vi "pic_step.vi"() -> ()   [LabVIEW 2018]
uses:
  Device VIs/Verbal.vi
  <vilib>/Instr/_visa.llb/VISA Configure Serial Port (Instr).vi
panel:
  in  "P3jog":bool caption="X jog"
  out "P3设定位置":i32
  in  "pic3位置":u16(ring) caption="位置" items=["位置0", "位置1", "位置2", "位置3"]
  in  "P3归0":bool
  in  "CH3启动":bool
  in  "CH3 运动步数":i32 caption="P3 步进"
  in  "Y 连续正转":bool
  in  "X连续反转":bool
  out "Yflag":bool
  out "0位":u8
  in  "P2 jog":bool caption="X jog"
  in  "P1jog":bool caption="X jog"
  in  "Zjog":bool caption="X jog"
  in  "Yjog":bool caption="X jog"
  in  "X jog":bool
  out "P2设定位置":i32
  out "P1设定位置":i32
  out "Z设定位置":i32
  out "Y设定位置":i32
  out "X设定位置":i32
  in  "pic2位置":u16(ring) caption="位置" items=["位置0", "位置1", "位置2", "位置3"]
  in  "pic1位置":u16(ring) caption="位置" items=["位置0", "位置1", "位置2", "位置3"]
  in  "Z轴位置":u16(ring) caption="位置" items=["位置0", "位置1", "位置2", "位置3"]
  in  "Y轴位置":u16(ring) caption="位置" items=["位置0", "位置1", "位置2", "位置3"]
  in  "X轴位置":u16(ring) caption="位置" items=["位置0", "位置1", "位置2", "位置3"]
  out "error in (no error)":errorcluster
  out "执行":bool
  in  "Z 归0":bool
  in  "Y 归0":bool
  in  "X 归0":bool
  out "当前位置":string[](array[string])
  in  "Z 连续反转":bool
  in  "Z 连续正转":bool
  in  "Y 连续反转":bool
  in  "X 连续正转":bool
  out "Z Left":bool caption="0位"
  out "Z Right":bool caption="限位"
  out "Y Left":bool caption="0位"
  out "Y Right":bool caption="限位"
  out "X Lift":bool caption="0位"
  out "X Right":bool caption="限位"
  in  "Z 启动":bool
  in  "Y 启动":bool
  in  "X 启动":bool
  in  "Step Z":i32 caption="Z 步进" min=-8388607 max=8388607
  in  "Step Y":i32 caption="Y 步进" min=-8388607 max=8388607
  in  "Step X":i32 caption="X 步进" min=-8388607 max=8388607
  in  "P2归0":bool
  in  "P1 归0":bool
  out "OK":bool
  in  "制动":bool
  in  "CH2启动":bool
  in  "CH1启动":bool
  in  "CH2 运动步数":i32 caption="P2 步进"
  in  "CH1 运动步数":i32 caption="P1 步进"
  out "CH2 当前位置":i32
  out "CH1 当前位置":i32
  out "状态":string
  out "error out":errorcluster
  # "X"
  # "Y"
  # "Z"
  # "P1"
  # "P2"
  # "P3"
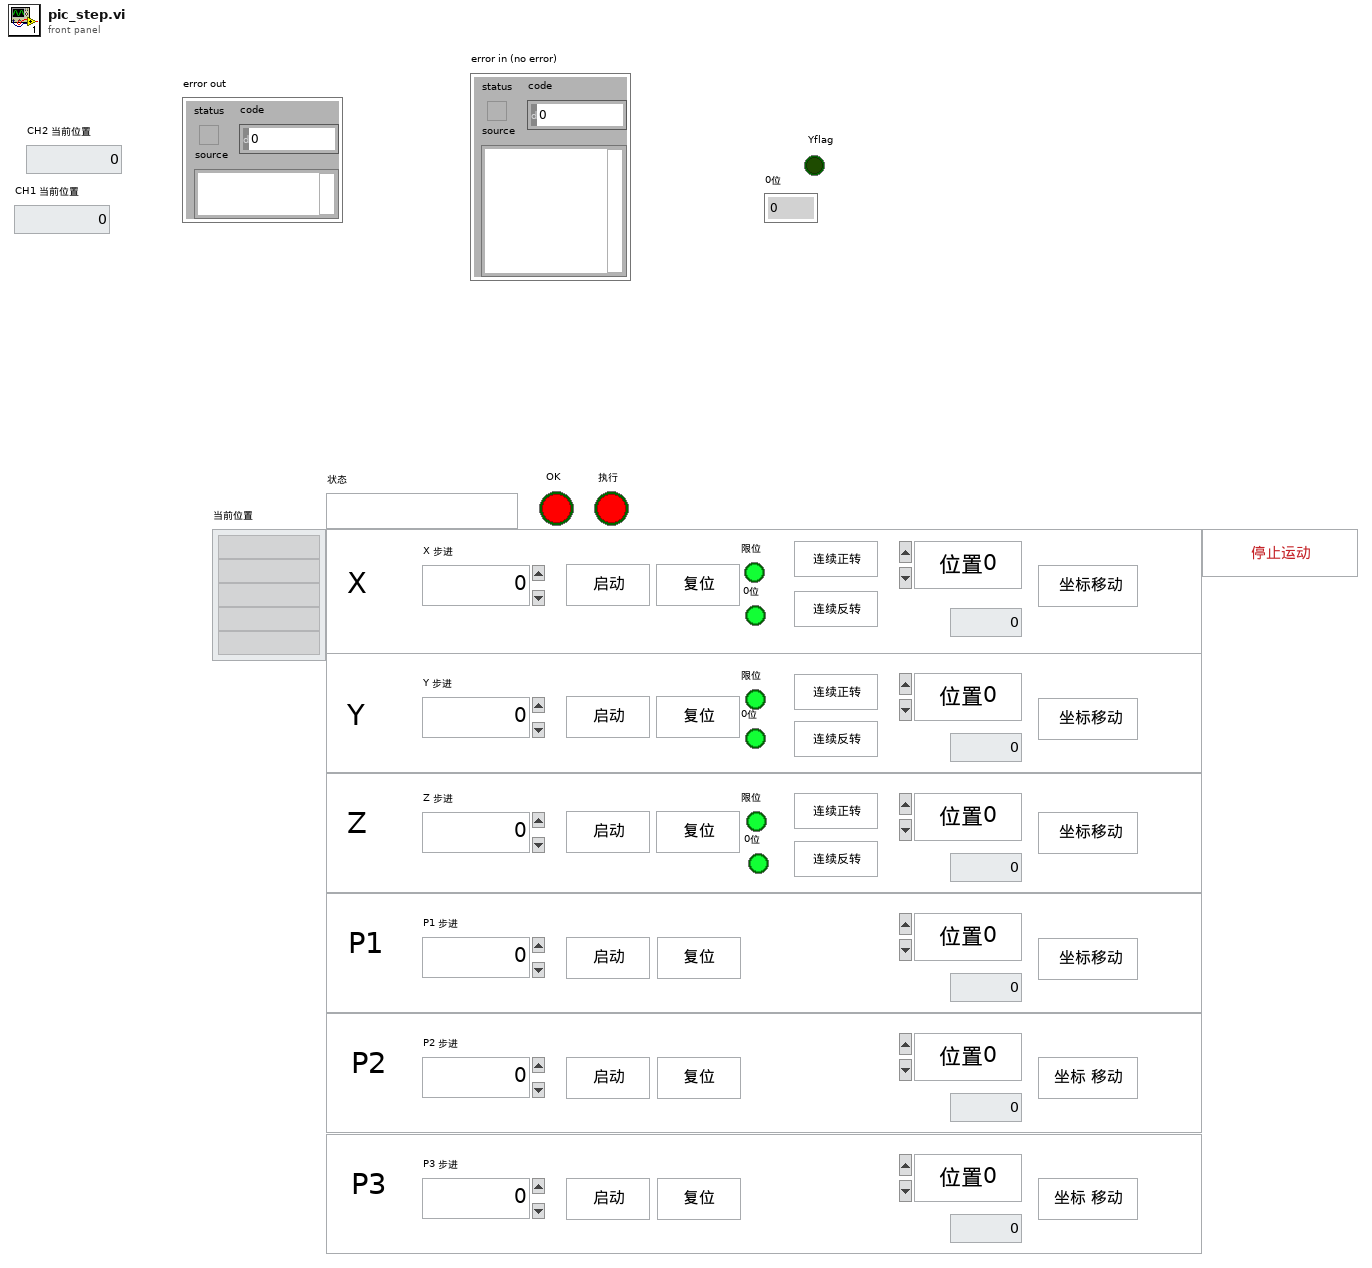
[diagram p1: front panel]
types:
  T1 = cluster{"DeviceKey":string, "Device Address":i32, "Controller Name":string}[]
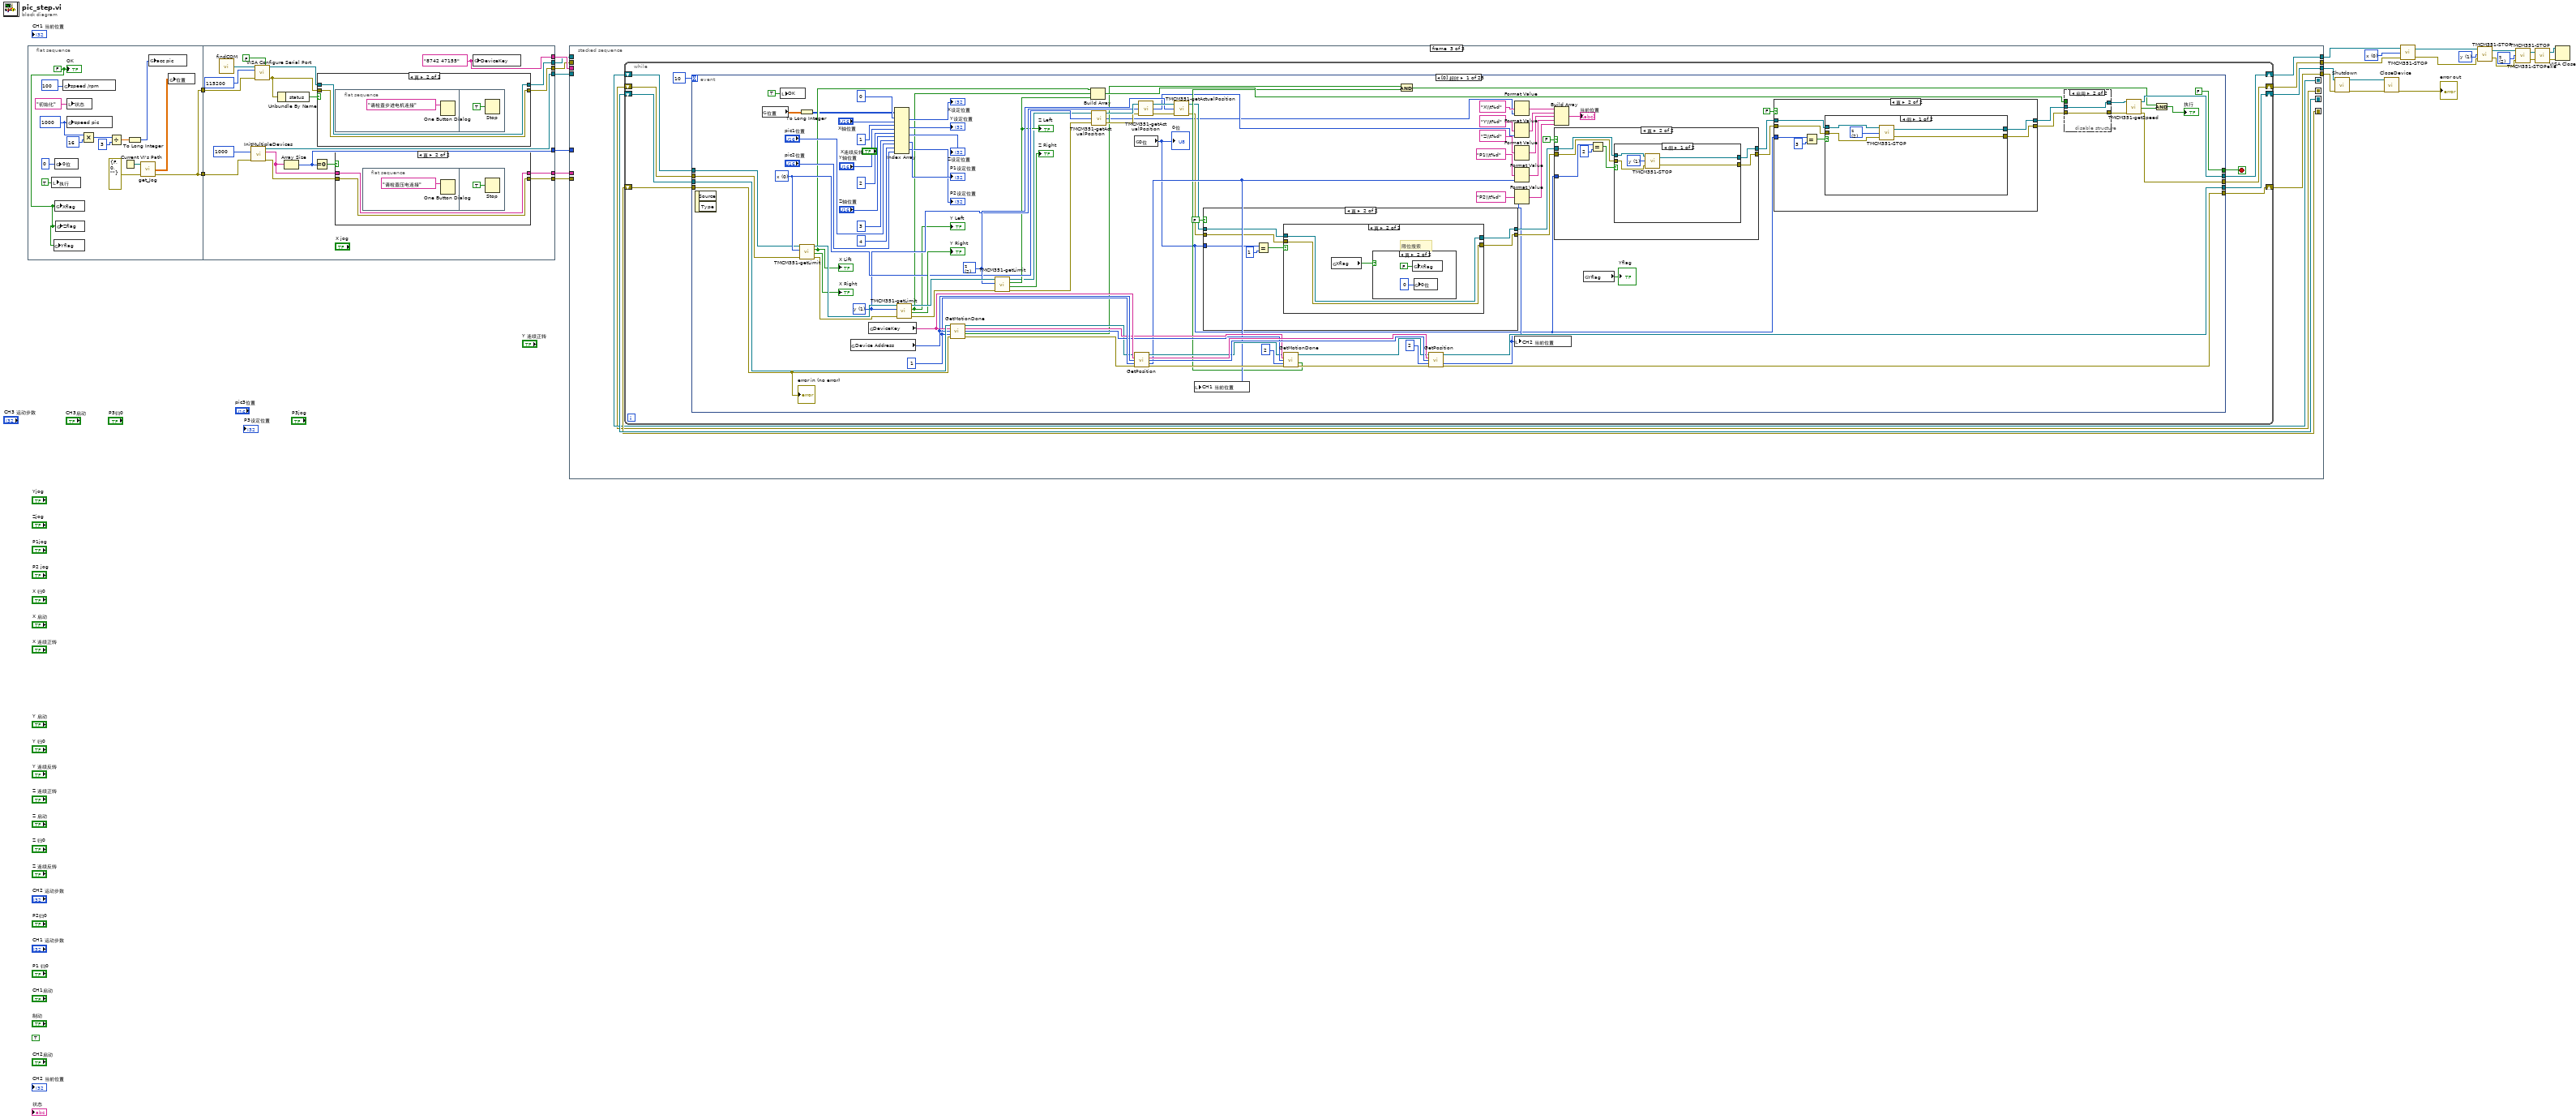
[diagram p0: block diagram]
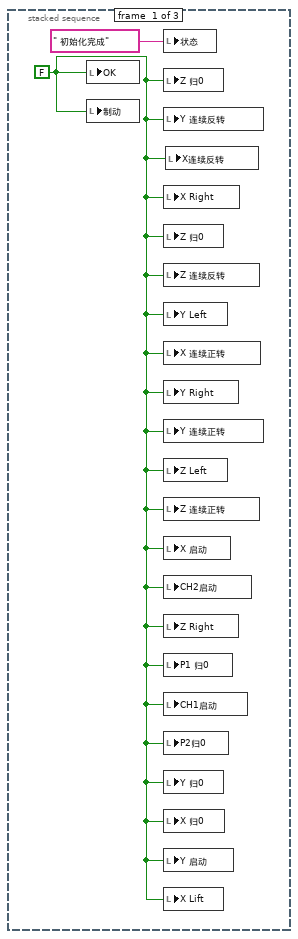
[diagram p4: hidden frame]
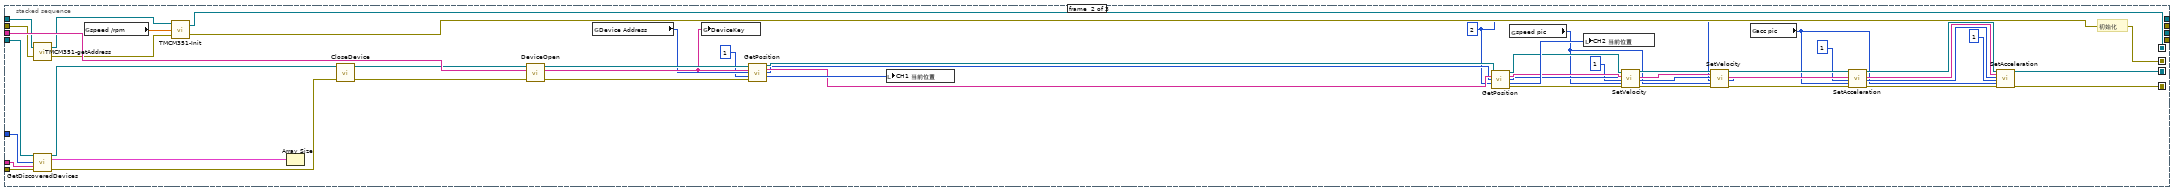
[diagram p5: hidden frame]
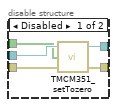
[diagram p6: hidden frame]
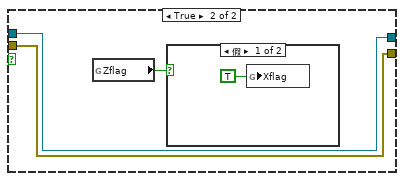
[diagram p8: hidden frame]
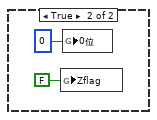
[diagram p9: hidden frame]
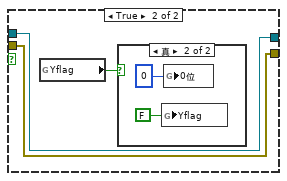
[diagram p11: hidden frame]
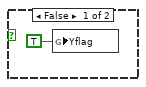
[diagram p12: hidden frame]
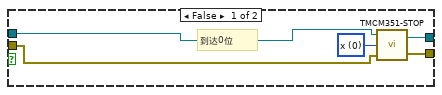
[diagram p14: hidden frame]
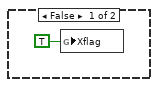
[diagram p15: hidden frame]
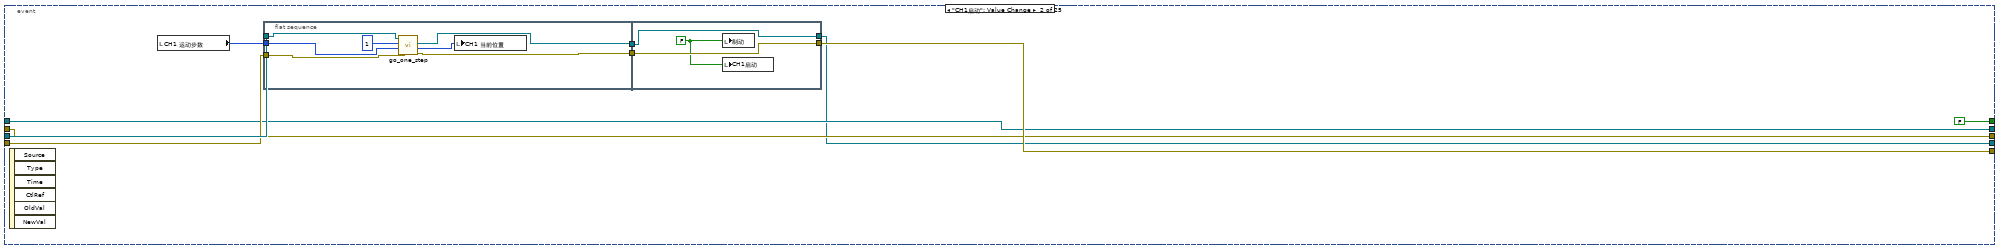
[diagram p16: hidden frame]
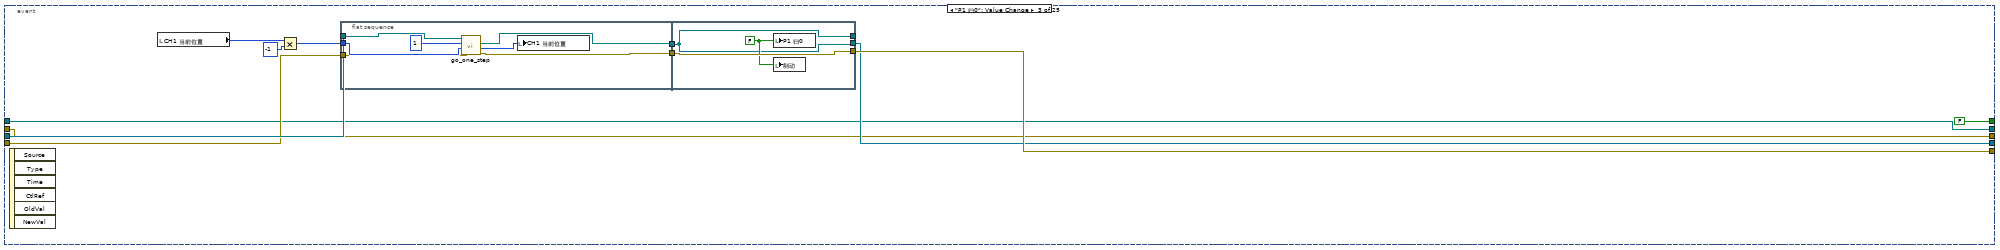
[diagram p17: hidden frame]
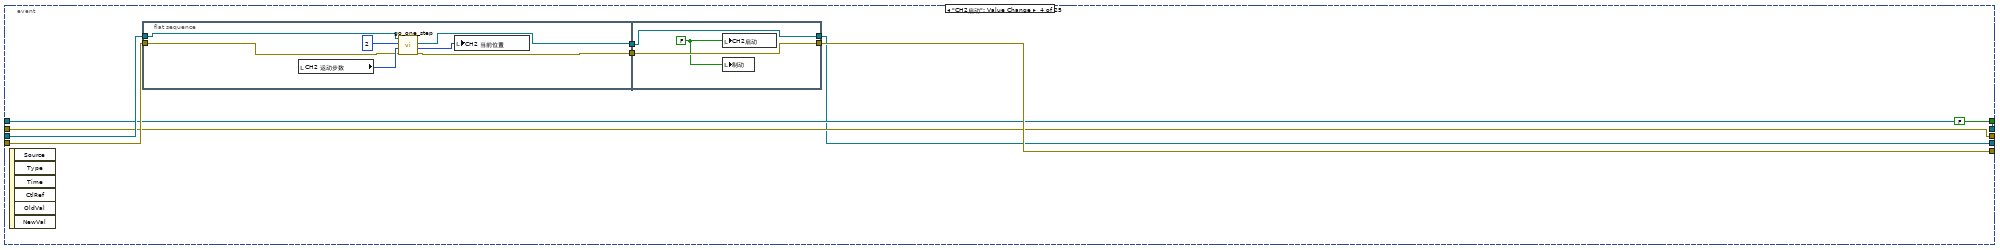
[diagram p18: hidden frame]
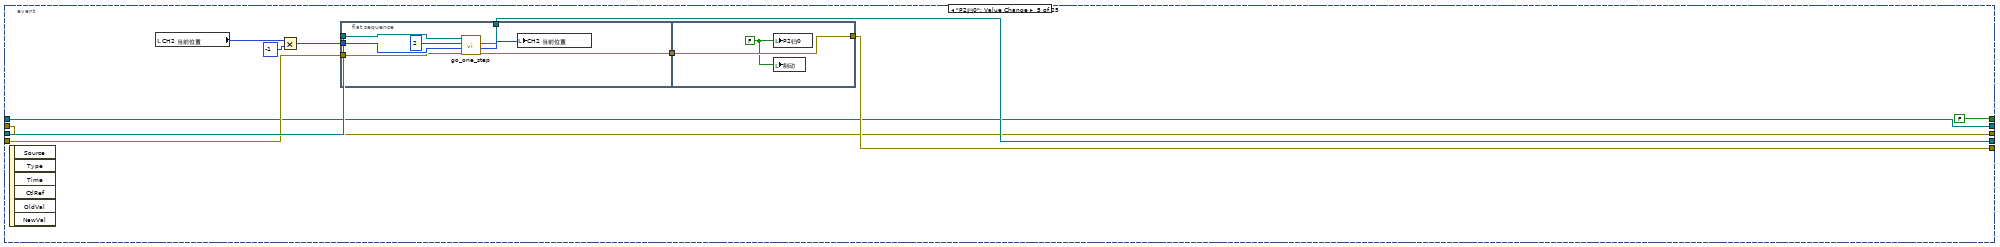
[diagram p19: hidden frame]
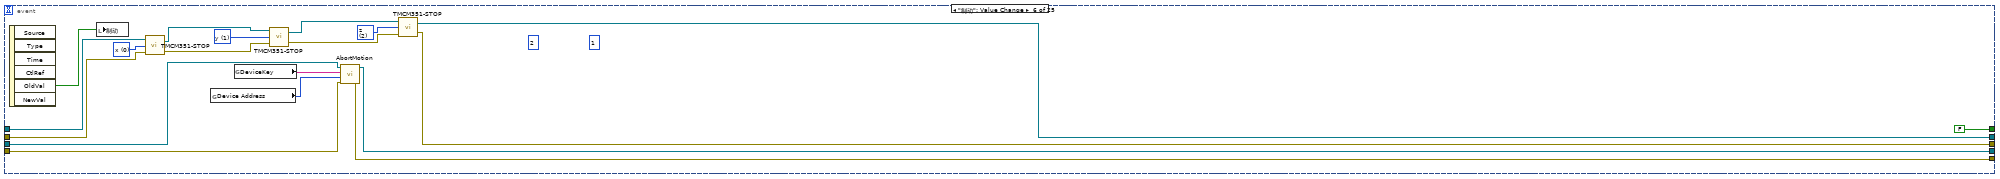
[diagram p20: hidden frame]
diagram:
  w10 = u8 2 items=["x", "y", "z"] ("motor")
  w11 = u8 1 items=["x", "y", "z"] ("motor")
  w12 = u8 0 items=["x", "y", "z"] ("motor")
  (unwired) TRUE
  n1 = flat-sequence {
    tunnel: [w31] -> w2
    tunnel: [w31] -> w1
    tunnel: [w61] -> w27
    tunnel: [w53] -> w26
    tunnel: [w52] -> w25
    tunnel: [w50] -> w24
    tunnel: [w49] -> w23
    tunnel: [w46] -> w22
    tunnel: [w45] -> w21
    tunnel: w2 -> [w44]
    tunnel: w1 -> [w43]
    frame #0 {
      w28 = FALSE ("OK")
      w37 = 1000 ("speed pic")
      n2 = local write "执行"(TRUE ("执行")) -> ()
      n3 = global write "Verbal.vi" "Yflag"(w28) -> ()
      n4 = global write "Verbal.vi" "0位"(u8 0 ("0位")) -> ()
      n5 = global write "Verbal.vi" "Xflag"(w28) -> ()
      n6 = global write "Verbal.vi" "Zflag"(w28) -> ()
      n7 = global write "Verbal.vi" "speed /rpm"(100 ("speed step")) -> ()
      n8 = local write "状态"("初始化" ("状态")) -> ()
      n9 = global write "Verbal.vi" "speed pic"(w37) -> ()
      n10 = Multiply(x=w37, y=u16 16) -> (x*y=w39:i32)
      n11 = Divide(x=w39, y=u16 3) -> (x/y=w36:dbl)
      n12 = Current VI's Path() -> (path=w33:path)
      n13 = To Long Integer(number=w36) -> (32bit integer=w35:i32)
      n14 = call "get_Jog.vi"("error in (no error)"=errorcluster {"status"=FALSE, "code"=0, "source"=""}, "路径"=w33) -> ("error out"=w31:errorcluster, "位置out"=w30:dbl[][])  [unwired: 2 in]
      n15 = global write "Verbal.vi" "acc pic"(w35) -> ()
      n16 = global write "Verbal.vi" "位置"(w30) -> ()
      "OK" <- w28
    }
    frame #1 {
      w61 = "8742 47155" ("Message")
      n17 = call "findCOM.vi"() -> ("VISA resource out"=w58:refnum<visa-resource-name>)  [unwired: 1 in]
      n18 = call "InitMultipleDevices.vi"("error in (no error)"=w43, "msecDelayForDiscovery"=1000) -> ("error out"=w47:errorcluster, "DeviceKey List Out"=w48:string[], "CmdLib Out"=w53:refnum<k24>)  [unwired: 3 in]
      n19 = call-poly "VISA Configure Serial Port"("VISA resource name"=w58, "Enable Termination\nChar (T)"=FALSE ("Enable Termination\nChar (T)"), "baud rate (9600)"=u32 115200, "error in (no error)"=w44) -> ("VISA resource name out"=w57:refnum<visa-resource-name>, "error out"=w55:errorcluster)  [unwired: 10 in]
      n20 = Unbundle By Name(w55) -> ("status"=w56:bool)
      n21 = Array Size(array=w48) -> (size(s)=w52:i32)
      n22 = Equal To 0?(x=w52) -> (x = 0?=w51:bool)
      n23 = case shown="真" w56 {
        tunnel: w57 -> [w69 w71]
        tunnel: w55 -> [w68 w70]
        tunnel: [w69 w71] -> w45
        tunnel: [w68 w70] -> w46
        frame False {
        }
        frame True {
          n24 = flat-sequence {
            frame #0 {
              n25 = One Button Dialog(message="请检查步进电机连接" ("消息")) -> ()  [unwired: 1 in, 1 out]
            }
            frame #1 {
              n26 = Stop(stop? (T)=TRUE ("停止？(T)")) -> ()
            }
          }
        }
      }
      n27 = case shown="真" w51 {
        tunnel: [w63 w65] -> w50
        tunnel: [w62 w64] -> w49
        tunnel: w48 -> [w63 w65]
        tunnel: w47 -> [w62 w64]
        frame False {
        }
        frame True {
          n28 = flat-sequence {
            frame #0 {
              n29 = One Button Dialog(message="请检查压电连接" ("消息")) -> ()  [unwired: 1 in, 1 out]
            }
            frame #1 {
              n30 = Stop(stop? (T)=TRUE ("停止？(T)")) -> ()
            }
          }
        }
      }
      n31 = global write "Verbal.vi" "DeviceKey"(w61) -> ()
    }
  }
  n32 = stacked-sequence {
    seq-local: [_ w79 _] -> [_ _ w134]
    seq-local: [_ w78 _] -> [_ _ w132]
    seq-local: [_ w119 _] -> [_ _ w131]
    seq-local: [_ w118 _] -> [_ _ w130]
    tunnel: w27 -> [_ w126 _]
    tunnel: [_ _ w133] -> w3
    tunnel: w25 -> [_ w125 _]
    tunnel: w24 -> [_ w124 _]
    tunnel: w26 -> [_ w123 _]
    tunnel: w23 -> [_ w122 _]
    tunnel: w22 -> [_ w121 _]
    tunnel: w21 -> [_ w120 _]
    tunnel: [_ _ w129] -> w14
    tunnel: [_ _ w128] -> w13
    tunnel: [_ _ w127] -> w4
    frame #0 {
      w74 = FALSE
      n33 = local write "OK"(w74) -> ()
      n34 = local write "制动"(w74) -> ()
      n35 = local write "状态"(" 初始化完成" ("Message")) -> ()
      n36 = local write "Z 归0"(w74) -> ()
      n37 = local write "Y 连续反转"(w74) -> ()
      n38 = local write "X Right"(w74) -> ()
      n39 = local write "Z 归0"(w74) -> ()
      n40 = local write "Z 连续反转"(w74) -> ()
      n41 = local write "Y Left"(w74) -> ()
      n42 = local write "X 连续正转"(w74) -> ()
      n43 = local write "Y Right"(w74) -> ()
      n44 = local write "Y 连续正转"(w74) -> ()
      n45 = local write "Z Left"(w74) -> ()
      n46 = local write "Z 连续正转"(w74) -> ()
      n47 = local write "X 启动"(w74) -> ()
      n48 = local write "CH2启动"(w74) -> ()
      n49 = local write "Z Right"(w74) -> ()
      n50 = local write "P1 归0"(w74) -> ()
      n51 = local write "CH1启动"(w74) -> ()
      n52 = local write "P2归0"(w74) -> ()
      n53 = local write "Y 归0"(w74) -> ()
      n54 = local write "X 归0"(w74) -> ()
      n55 = local write "Y 启动"(w74) -> ()
      n56 = local write "X Lift"(w74) -> ()
      n57 = local write "X连续反转"(w74) -> ()
    }
    frame #1 {
      w94 = 2 ("Motor")
      # "初始化"
      n58 = call "TMCM351-getAddress.vi"("错误输入"=w121, "com in"=w120) -> ("错误输出"=w92:errorcluster, "com out"=w77:refnum<visa-resource-name>)
      n59 = call "GetDiscoveredDevices.vi"("CmdLib In"=w123, "Master Count"=w125, "DeviceKey List"=w124, "error in"=w122) -> ("CmdLib Out"=w116:refnum<k24>, "Device Array"=w117:T1, "error out"=w114:errorcluster)  [unwired: 9 in]
      n60 = global read "Verbal.vi" "speed /rpm"() -> (w76:dbl)
      n61 = call "TMCM351-Init.vi"("错误输入"=w92, "Speed /rpm"=w76, "com in"=w77) -> ("错误输出"=w118:errorcluster, "com out"=w119:refnum<visa-resource-name>)
      n62 = Array Size(array=w117) -> ()  [unwired: 1 out]
      n63 = call "CloseDevice.vi"("error in"=w114, "CmdLib In"=w116) -> ("error out"=w113:errorcluster, "CmdLib Out"=w115:refnum<k24>)  [unwired: 8 in]
      n64 = call "DeviceOpen.vi"("error in (no error)"=w113, "DeviceKey In"=w126, "CmdLib In"=w115) -> ("error out"=w108:errorcluster, "DeviceKey Out"=w111:string, "CmdLib Out"=w112:refnum<k24>)  [unwired: 2 in]
      n65 = global read "Verbal.vi" "Device Address"() -> (w110:i32)
      n66 = global write "Verbal.vi" "DeviceKey"(w111) -> ()
      n67 = call "GetPosition.vi"("CmdLib In"=w112, "DeviceKey In"=w111, "Device Address In"=w110, "Motor"=1, "error in (no error)"=w108) -> ("CmdLib Out"=w106:refnum<k24>, "DeviceKey Out"=w105:string, "Device Address Out"=w104:i32, "Position"=w107:i32)  [unwired: 6 in, 1 out]
      n68 = local write "CH1 当前位置"(w107) -> ()
      n69 = call "GetPosition.vi"("CmdLib In"=w106, "DeviceKey In"=w105, "Device Address In"=w104, "Motor"=w94) -> ("CmdLib Out"=w102:refnum<k24>, "DeviceKey Out"=w101:string, "Device Address Out"=w100:i32, "Position"=w103:i32, "error out"=w98:errorcluster)  [unwired: 7 in]
      n70 = global read "Verbal.vi" "speed pic"() -> (w91:i32)
      n71 = local write "CH2 当前位置"(w103) -> ()
      n72 = call "SetVelocity.vi"("CmdLib In"=w102, "DeviceKey In"=w101, "Device Address In"=w100, "Motor"=1, "Steps Per Sec"=w91, "error in (no error)"=w98) -> ("CmdLib Out"=w97:refnum<k24>, "DeviceKey Out"=w96:string, "Device Address Out"=w95:i32, "error out"=w93:errorcluster)  [unwired: 10 in]
      n73 = call "SetVelocity.vi"("CmdLib In"=w97, "DeviceKey In"=w96, "Device Address In"=w95, "Motor"=w94, "Steps Per Sec"=w91, "error in (no error)"=w93) -> ("CmdLib Out"=w90:refnum<k24>, "DeviceKey Out"=w89:string, "Device Address Out"=w88:i32, "error out"=w86:errorcluster)  [unwired: 10 in]
      n74 = global read "Verbal.vi" "acc pic"() -> (w81:i32)
      n75 = call "SetAcceleration.vi"("CmdLib In"=w90, "DeviceKey In"=w89, "Device Address In"=w88, "Motor"=1, "Steps Per Sec 2"=w81, "error in (no error)"=w86) -> ("CmdLib Out"=w85:refnum<k24>, "DeviceKey Out"=w84:string, "Device Address Out"=w83:i32, "error out"=w80:errorcluster)  [unwired: 10 in]
      n76 = call "SetAcceleration.vi"("CmdLib In"=w85, "DeviceKey In"=w84, "Device Address In"=w83, "Motor"=1, "Steps Per Sec 2"=w81, "error in (no error)"=w80) -> ("CmdLib Out"=w79:refnum<k24>, "error out"=w78:errorcluster)  [unwired: 10 in, 2 out]
    }
    frame #2 {
      n77 = while {
        shift-right: [w142] -> w133
        shift-left: w132 -> [w140]
        shift-right: [w139] -> w127
        shift-left: w134 -> [w143]
        shift-right: [w138] -> w129
        shift-left: w131 -> [w136]
        shift-right: [w137] -> w128
        shift-left: w130 -> [w135]
        stop <- w141 stop-if-true
        n78 = event shown="[0] 超时" {
          selector: _ -> [_ _ _ _ _ _ _ _ _ _ _ _ _ _ _ _ _ _ _ _ _ _ _ _ _]
          dyn-events: _ -> [_ _ _ _ _ _ _ _ _ _ _ _ _ _ _ _ _ _ _ _ _ _ _ _ _]
          timeout: 10 -> [_ _ _ _ _ _ _ _ _ _ _ _ _ _ _ _ _ _ _ _ _ _ _ _ _]
          tunnel: w143 -> [w236 w318 w337 w359 w377 w406 w424 w440 w445 w458 w469 w484 w522 w561 w590 w601 w612 w623 w634 w645 w656 w666 w676 w694 w706]
          tunnel: w140 -> [w188 w317 w336 w357 w376 w407 w423 w439 w444 w457 w468 w483 w521 w560 w589 w600 w611 w622 w633 w644 w655 w665 w675 w689 w701]
          tunnel: [w237 w316 w334 w358 w375 w392 w422 w438 w444 w457 w468 w483 w521 w560 w589 w600 w611 w622 w633 w644 w655 w665 w675 w687 w699] -> w142
          tunnel: [FALSE FALSE FALSE FALSE FALSE FALSE TRUE TRUE FALSE FALSE FALSE FALSE FALSE _ _ _ _ _ _ _ _ _ _ _ _] -> w141
          tunnel: w136 -> [w164 w312 w330 w354 w371 w404 w413 w428 w450 w461 w473 w478 w514 w554 w599 w607 w618 w629 w640 w651 w662 w672 w682 w686 w698]
          tunnel: w135 -> [w163 w311 w329 w353 w370 w403 w412 w427 w449 w460 w471 w475 w513 w553 w598 w606 w617 w628 w639 w650 w661 w671 w681 w685 w697]
          tunnel: [w203 w309 w331 w351 w372 w391 w409 w436 w445 w458 w469 w484 w522 w561 w590 w601 w612 w623 w634 w645 w656 w666 w676 w688 w700] -> w139
          tunnel: [w185 w312 w330 w354 w371 w395 w411 w426 w447 w456 w467 w477 w520 w558 w594 w605 w616 w627 w638 w649 w660 w668 w678 w686 w698] -> w138
          tunnel: [w184 w311 w329 w353 w370 w394 w410 w425 w446 w455 w466 w476 w519 w559 w593 w604 w615 w626 w637 w648 w659 w667 w677 w685 w697] -> w137
          event Timeout {
            w210 = u8 2 items=["x", "y", "z"] ("motor")
            w191 = u8 1 items=["x", "y", "z"] ("motor")
            w192 = u8 0 items=["x", "y", "z"] ("motor")
            w233 = 1 ("Motor")
            n79 = event-data() -> ()  [unwired: 1 in, 2 out]
            n80 = global read "Verbal.vi" "位置"() -> (w159:dbl[][])
            n81 = local write "OK"(TRUE ("等待指令")) -> ()
            n82 = To Long Integer(number=w159) -> (32bit integer=w158:i32[][])
            n83 = call "TMCM351-getLimit.vi"("错误输入"=w163, "motor"=w192, "com in"=w164) -> ("错误输出"=w213:errorcluster, "right limit"=→"X Right":bool, "left limit"=w162:bool, "com out"=w214:refnum<visa-resource-name>)  [unwired: 1 in]
            "X Lift" <- w162
            n84 = global read "Verbal.vi" "Device Address"() -> (w234:i32)
            n85 = global read "Verbal.vi" "DeviceKey"() -> (w235:string)
            n86 = Index Array(array=w158, index (row) #1=0 ("索引 (行)"), index (col) #1="X轴位置", index (row) #2=1 ("索引 (行)"), index (col) #2="Y轴位置", index (row) #3=2 ("索引 (行)"), index (col) #3="Z轴位置", index (row) #4=3 ("索引 (行)"), index (col) #4="pic1位置", index (row) #5=4 ("索引 (行)"), index (col) #5="pic2位置") -> (element #1=→"X设定位置":i32, element #2=→"Y设定位置":i32, element #3=→"Z设定位置":i32, element #4=→"P1设定位置":i32, element #5=→"P2设定位置":i32)
            n87 = call "TMCM351-getLimit.vi"("错误输入"=w213, "motor"=w191, "com in"=w214) -> ("错误输出"=w211:errorcluster, "right limit"=→"Y Right":bool, "left limit"=w161:bool, "com out"=w212:refnum<visa-resource-name>)  [unwired: 1 in]
            "Y Left" <- w161
            n88 = call "GetMotionDone.vi"("CmdLib In"=w236, "DeviceKey In"=w235, "Device Address In"=w234, "Motor"=w233, "error in (no error)"=w188) -> ("CmdLib Out"=w208:refnum<k24>, "DeviceKey Out"=w232:string, "Device Address Out"=w231:i32, "Is Motion Done"=w190:bool, "error out"=w209:errorcluster)  [unwired: 6 in]
            n89 = call "TMCM351-getLimit.vi"("错误输入"=w211, "motor"=w210, "com in"=w212) -> ("错误输出"=w156:errorcluster, "right limit"=→"Z Right":bool, "left limit"=w160:bool, "com out"=w157:refnum<visa-resource-name>)  [unwired: 1 in]
            "Z Left" <- w160
            n90 = Build Array(w162, w161, w160) -> (w195:bool[])
            n91 = call "TMCM351-getActualPosition.vi"("错误输入"=w156, "motor"=w192, "com in"=w157) -> ("错误输出"=w228:errorcluster, "Pisotion"=w150:i32, "com out"=w229:refnum<visa-resource-name>)
            n92 = global read "Verbal.vi" "0位"() -> (w149:u8)
            "0位" <- w149
            n93 = call "GetPosition.vi"("CmdLib In"=w208, "DeviceKey In"=w235, "Device Address In"=w234, "Motor"=w233, "error in (no error)"=w209) -> ("CmdLib Out"=w207:refnum<k24>, "DeviceKey Out"=w241:string, "Device Address Out"=w240:i32, "Position"=w194:i32, "error out"=w206:errorcluster)  [unwired: 6 in]
            n94 = call "TMCM351-getActualPosition.vi"("错误输入"=w228, "motor"=w191, "com in"=w229) -> ("错误输出"=w226:errorcluster, "Pisotion"=w151:i32, "com out"=w227:refnum<visa-resource-name>)
            n95 = call "TMCM351-getActualPosition.vi"("错误输入"=w226, "motor"=w210, "com in"=w227) -> ("错误输出"=w154:errorcluster, "com out"=w155:refnum<visa-resource-name>)  [unwired: 1 out]
            n96 = local write "CH1 当前位置"(w194) -> ()
            n97 = case shown="真" FALSE {
              tunnel: [w290 w297] -> w202
              tunnel: [w289 w296] -> w201
              tunnel: w155 -> [w290 w295]
              tunnel: w154 -> [w289 w294]
              tunnel: w149 -> [_ w293]
              frame False {
              }
              frame True {
                n98 = Equal?(x=w293, y=1) -> (x = y?=w291:bool)
                n99 = case shown="真" w291 {
                  tunnel: w295 -> [w301 w305]
                  tunnel: w294 -> [w300 w304]
                  tunnel: [w299 w305] -> w297
                  tunnel: [w298 w304] -> w296
                  frame False {
                    w302 = u8 0 items=["x", "y", "z"] ("motor")
                    # "到达0位"
                    n100 = call "TMCM351-STOP.vi"("错误输入"=w300, "motor"=w302, "com in"=w301) -> ("错误输出"=w298:errorcluster, "com out"=w299:refnum<visa-resource-name>)
                  }
                  frame True {
                    # "限位搜索"
                    n101 = global read "Verbal.vi" "Xflag"() -> (w303:bool)
                    n102 = case shown="真" w303 {
                      frame False {
                        n103 = global write "Verbal.vi" "Xflag"(TRUE ("Xflag")) -> ()
                      }
                      frame True {
                        n104 = global write "Verbal.vi" "Xflag"(FALSE ("Xflag")) -> ()
                        n105 = global write "Verbal.vi" "0位"(u8 0 ("0位")) -> ()
                      }
                    }
                  }
                }
              }
            }
            n106 = call "GetMotionDone.vi"("CmdLib In"=w207, "DeviceKey In"=w232, "Device Address In"=w231, "Motor"=2, "error in (no error)"=w206) -> ("CmdLib Out"=w205:refnum<k24>, "Is Motion Done"=w189:bool, "error out"=w204:errorcluster)  [unwired: 6 in, 2 out]
            n107 = And(x=w190, y=w189) -> (x .and. y?=w183:bool)
            n108 = call "GetPosition.vi"("CmdLib In"=w205, "DeviceKey In"=w241, "Device Address In"=w240, "Motor"=2, "error in (no error)"=w204) -> ("CmdLib Out"=w203:refnum<k24>, "Position"=w193:i32, "error out"=w237:errorcluster)  [unwired: 6 in, 2 out]
            n109 = Format Value(format string="X\\t%d" ("格式字符串"), value (0)=w150) -> (output string=w220:string)  [unwired: 1 in]
            n110 = Format Value(format string="Y\\t%d" ("格式字符串"), value (0)=w151) -> (output string=w219:string)  [unwired: 1 in]
            n111 = Format Value(format string="Z\\t%d" ("格式字符串")) -> (output string=w218:string)  [unwired: 2 in]
            n112 = Format Value(format string="P1\\t%d" ("格式字符串"), value (0)=w194) -> (output string=w217:string)  [unwired: 1 in]
            n113 = Format Value(format string="P2\\t%d" ("格式字符串"), value (0)=w193) -> (output string=w216:string)  [unwired: 1 in]
            n114 = local write "CH2 当前位置"(w193) -> ()
            n115 = Build Array(w220, w219, w218, w217, w216) -> (→"当前位置":string[])
            n116 = case shown="真" FALSE {
              tunnel: w202 -> [w270 w277]
              tunnel: w201 -> [w269 w276]
              tunnel: [w270 w275] -> w200
              tunnel: [w269 w274] -> w199
              tunnel: w149 -> [_ w273]
              frame False {
              }
              frame True {
                n117 = Equal?(x=w273, y=u8 2) -> (x = y?=w271:bool)
                n118 = case shown="假" w271 {
                  tunnel: w277 -> [w281 w285]
                  tunnel: w276 -> [w280 w284]
                  tunnel: [w279 w285] -> w275
                  tunnel: [w278 w284] -> w274
                  frame False {
                    w282 = u8 1 items=["x", "y", "z"] ("motor")
                    n119 = call "TMCM351-STOP.vi"("错误输入"=w280, "motor"=w282, "com in"=w281) -> ("错误输出"=w278:errorcluster, "com out"=w279:refnum<visa-resource-name>)
                  }
                  frame True {
                    n120 = global read "Verbal.vi" "Yflag"() -> (w283:bool)
                    n121 = case shown="真" w283 {
                      frame False {
                        n122 = global write "Verbal.vi" "Yflag"(TRUE) -> ()
                      }
                      frame True {
                        n123 = global write "Verbal.vi" "Yflag"(FALSE) -> ()
                        n124 = global write "Verbal.vi" "0位"(u8 0 ("0位")) -> ()
                      }
                    }
                  }
                }
              }
            }
            n125 = global read "Verbal.vi" "Yflag"() -> (→"Yflag":bool)
            n126 = case shown="真" FALSE {
              tunnel: w200 -> [w250 w257]
              tunnel: w199 -> [w249 w256]
              tunnel: [w250 w255] -> w153
              tunnel: [w249 w254] -> w152
              tunnel: w149 -> [_ w253]
              frame False {
              }
              frame True {
                n127 = Equal?(x=w253, y=u8 3) -> (x = y?=w251:bool)
                n128 = case shown="假" w251 {
                  tunnel: w257 -> [w261 w265]
                  tunnel: w256 -> [w260 w264]
                  tunnel: [w259 w265] -> w255
                  tunnel: [w258 w264] -> w254
                  frame False {
                    w262 = u8 2 items=["x", "y", "z"] ("motor")
                    n129 = call "TMCM351-STOP.vi"("错误输入"=w260, "motor"=w262, "com in"=w261) -> ("错误输出"=w258:errorcluster, "com out"=w259:refnum<visa-resource-name>)
                  }
                  frame True {
                    n130 = global read "Verbal.vi" "Zflag"() -> (w263:bool)
                    n131 = case shown="假" w263 {
                      frame False {
                        n132 = global write "Verbal.vi" "Xflag"(TRUE ("Xflag")) -> ()
                      }
                      frame True {
                        n133 = global write "Verbal.vi" "Zflag"(FALSE ("Zflag")) -> ()
                        n134 = global write "Verbal.vi" "0位"(u8 0 ("0位")) -> ()
                      }
                    }
                  }
                }
              }
            }
            n135 = disable-structure shown="启用" {
              disable-tunnel: w153 -> [w246 w248]
              disable-tunnel: w152 -> [w245 w247]
              disable-tunnel: w195 -> [w244 _]
              disable-tunnel: [w243 w248] -> w187
              disable-tunnel: [w242 w247] -> w186
              frame Disabled {
                n136 = call "TMCM351_setTozero.vi"("错误输入"=w245, "归0到位"=w244, "com in"=w246) -> ("错误输出"=w242:errorcluster, "com out"=w243:refnum<visa-resource-name>)  [unwired: 1 in]
              }
              frame Enabled {
              }
            }
            n137 = call "TMCM351-getSpeed.vi"("错误输入"=w186, "com in"=w187) -> ("错误输出"=w184:errorcluster, "Motion Done"=w182:bool, "com out"=w185:refnum<visa-resource-name>)  [unwired: 2 in, 1 out]
            n138 = And(x=w183, y=w182) -> (x .and. y?=→"执行":bool)
            "error in (no error)" <- w188
          }
          event "CH1启动": Value Change {
            n139 = event-data() -> ()  [unwired: 1 in, 6 out]
            n140 = local read "CH1 运动步数"() -> (w314:i32)
            n141 = flat-sequence {
              tunnel: w318 -> [w325]
              tunnel: w317 -> [w324]
              tunnel: w314 -> [w322]
              tunnel: [w323] -> w313
              tunnel: [w319] -> w310
              tunnel: [w328] -> w316
              tunnel: w313 -> [w328]
              tunnel: [w326] -> w309
              tunnel: w310 -> [w326]
              frame #0 {
                n142 = call "go_one_step.vi"("error in"=w324, "Step"=w322, "Motor"=1, "CmdLib In"=w325) -> ("error out"=w323:errorcluster, "Position"=w320:i32, "CmdLib Out"=w319:refnum<k24>)  [unwired: 1 in]
                n143 = local write "CH1 当前位置"(w320) -> ()
              }
              frame #1 {
                w327 = FALSE ("制动")
                n144 = local write "制动"(w327) -> ()
                n145 = local write "CH1启动"(w327) -> ()
              }
            }
          }
          event "P1 归0": Value Change {
            n146 = event-data() -> ()  [unwired: 1 in, 6 out]
            n147 = local read "CH1 当前位置"() -> (w340:i32)
            n148 = Multiply(x=w340, y=-1) -> (x*y=w338:i32)
            n149 = flat-sequence {
              tunnel: w338 -> [w347]
              tunnel: w337 -> [w346]
              tunnel: w336 -> [w345]
              tunnel: [w344] -> w333
              tunnel: [w341] -> w332
              tunnel: [w350] -> w334
              tunnel: w333 -> [w350]
              tunnel: [w348] -> _
              tunnel: w332 -> [w348]
              tunnel: [w348] -> w331
              frame #0 {
                n150 = call "go_one_step.vi"("error in"=w345, "Step"=w347, "Motor"=1, "CmdLib In"=w346) -> ("error out"=w344:errorcluster, "Position"=w342:i32, "CmdLib Out"=w341:refnum<k24>)  [unwired: 1 in]
                n151 = local write "CH1 当前位置"(w342) -> ()
              }
              frame #1 {
                w349 = FALSE ("制动")
                n152 = local write "P1 归0"(w349) -> ()
                n153 = local write "制动"(w349) -> ()
              }
            }
          }
          event "CH2启动": Value Change {
            n154 = event-data() -> ()  [unwired: 1 in, 6 out]
            n155 = flat-sequence {
              tunnel: w359 -> [w366]
              tunnel: w357 -> [w363]
              tunnel: [w364] -> w355
              tunnel: [w360] -> w352
              tunnel: [w369] -> w358
              tunnel: w355 -> [w369]
              tunnel: [w367] -> w351
              tunnel: w352 -> [w367]
              frame #0 {
                n156 = local read "CH2 运动步数"() -> (w365:i32)
                n157 = call "go_one_step.vi"("error in"=w363, "Step"=w365, "Motor"=2, "CmdLib In"=w366) -> ("error out"=w364:errorcluster, "Position"=w361:i32, "CmdLib Out"=w360:refnum<k24>)  [unwired: 1 in]
                n158 = local write "CH2 当前位置"(w361) -> ()
              }
              frame #1 {
                w368 = FALSE
                n159 = local write "CH2启动"(w368) -> ()
                n160 = local write "制动"(w368) -> ()
              }
            }
          }
          event "P2归0": Value Change {
            n161 = event-data() -> ()  [unwired: 1 in, 6 out]
            n162 = local read "CH2 当前位置"() -> (w380:i32)
            n163 = Multiply(x=w380, y=-1) -> (x*y=w378:i32)
            n164 = flat-sequence {
              tunnel: w378 -> [w387]
              tunnel: w377 -> [w386]
              tunnel: w376 -> [w385]
              tunnel: [w384] -> w373
              tunnel: [w381] -> w372
              tunnel: [w389] -> w375
              tunnel: w373 -> [w389]
              frame #0 {
                n165 = call "go_one_step.vi"("error in"=w385, "Step"=w387, "Motor"=2, "CmdLib In"=w386) -> ("error out"=w384:errorcluster, "Position"=w382:i32, "CmdLib Out"=w381:refnum<k24>)  [unwired: 1 in]
                n166 = local write "CH2 当前位置"(w382) -> ()
              }
              frame #1 {
                w388 = FALSE ("制动")
                n167 = local write "P2归0"(w388) -> ()
                n168 = local write "制动"(w388) -> ()
              }
            }
          }
          event "制动": Value Change {
            w396 = u8 2 items=["x", "y", "z"] ("motor")
            w399 = u8 1 items=["x", "y", "z"] ("motor")
            w402 = u8 0 items=["x", "y", "z"] ("motor")
            (unwired) 2 ("Motor")
            (unwired) 1 ("Motor")
            n169 = event-data() -> ("OldVal"=w390:bool)  [unwired: 1 in, 5 out]
            n170 = local write "制动"(w390) -> ()
            n171 = call "TMCM351-STOP.vi"("错误输入"=w403, "motor"=w402, "com in"=w404) -> ("错误输出"=w400:errorcluster, "com out"=w401:refnum<visa-resource-name>)
            n172 = global read "Verbal.vi" "Device Address"() -> (w393:i32)
            n173 = global read "Verbal.vi" "DeviceKey"() -> (w405:string)
            n174 = call "TMCM351-STOP.vi"("错误输入"=w400, "motor"=w399, "com in"=w401) -> ("错误输出"=w397:errorcluster, "com out"=w398:refnum<visa-resource-name>)
            n175 = call "AbortMotion.vi"("error in (no error)"=w407, "Device Address In"=w393, "DeviceKey In"=w405, "CmdLib In"=w406) -> ("error out"=w392:errorcluster, "CmdLib Out"=w391:refnum<k24>)  [unwired: 2 out]
            n176 = call "TMCM351-STOP.vi"("错误输入"=w397, "motor"=w396, "com in"=w398) -> ("错误输出"=w394:errorcluster, "com out"=w395:refnum<visa-resource-name>)
          }
          event Application Instance Close {
            w414 = u8 2 items=["x", "y", "z"] ("motor")
            w415 = u8 1 items=["x", "y", "z"] ("motor")
            w420 = u8 0 items=["x", "y", "z"] ("motor")
            n177 = event-data() -> ()  [unwired: 1 in, 4 out]
            n178 = call "Shutdown.vi"("error in (no error)"=w423, "CmdLib In"=w424) -> ("error out"=w422:errorcluster, "CmdLib Out"=w409:refnum<k24>)  [unwired: 4 in]
            n179 = call "TMCM351-STOP.vi"("错误输入"=w412, "motor"=w420, "com in"=w413) -> ("错误输出"=w419:errorcluster, "com out"=w418:refnum<visa-resource-name>)
            n180 = call "TMCM351-STOP.vi"("错误输入"=w419, "motor"=w415, "com in"=w418) -> ("错误输出"=w417:errorcluster, "com out"=w416:refnum<visa-resource-name>)
            n181 = call "TMCM351-STOP.vi"("错误输入"=w417, "motor"=w414, "com in"=w416) -> ("错误输出"=w410:errorcluster, "com out"=w411:refnum<visa-resource-name>)
          }
          event Panel Close {
            w429 = u8 2 items=["x", "y", "z"] ("motor")
            w430 = u8 1 items=["x", "y", "z"] ("motor")
            w435 = u8 0 items=["x", "y", "z"] ("motor")
            n182 = event-data() -> ()  [unwired: 1 in, 4 out]
            n183 = call "Shutdown.vi"("error in (no error)"=w439, "CmdLib In"=w440) -> ("error out"=w438:errorcluster, "CmdLib Out"=w436:refnum<k24>)  [unwired: 4 in]
            n184 = call "TMCM351-STOP.vi"("错误输入"=w427, "motor"=w435, "com in"=w428) -> ("错误输出"=w434:errorcluster, "com out"=w433:refnum<visa-resource-name>)
            n185 = call "TMCM351-STOP.vi"("错误输入"=w434, "motor"=w430, "com in"=w433) -> ("错误输出"=w432:errorcluster, "com out"=w431:refnum<visa-resource-name>)
            n186 = call "TMCM351-STOP.vi"("错误输入"=w432, "motor"=w429, "com in"=w431) -> ("错误输出"=w425:errorcluster, "com out"=w426:refnum<visa-resource-name>)
          }
          event "X 启动": Value Change {
            w451 = u8 0 items=["x", "y", "z"] ("motor")
            n187 = event-data() -> ("CtlRef"=w442:refnum<vi>, "OldVal"=w441:bool)  [unwired: 1 in, 4 out]
            n188 = property class="Bool (严格)"(reference=w442, "Value"=w441) -> ()  [unwired: 1 in, 2 out]
            n189 = call "TMCM351-Step.vi"("错误输入"=w449, "Step"="Step X", "motor"=w451, "com in"=w450) -> ("错误输出"=w446:errorcluster, "com out"=w447:refnum<visa-resource-name>)  [unwired: 2 in]
          }
          event "Y 启动": Value Change {
            w462 = u8 1 items=["x", "y", "z"] ("motor")
            n190 = event-data() -> ("CtlRef"=w453:refnum<vi>, "OldVal"=w452:bool)  [unwired: 1 in, 4 out]
            n191 = property class="Bool (严格)"(reference=w453, "Value"=w452) -> ()  [unwired: 1 in, 2 out]
            n192 = call "TMCM351-Step.vi"("错误输入"=w460, "Step"="Step Y", "motor"=w462, "com in"=w461) -> ("错误输出"=w455:errorcluster, "com out"=w456:refnum<visa-resource-name>)  [unwired: 2 in]
          }
          event "Z 启动": Value Change {
            w472 = u8 2 items=["x", "y", "z"] ("motor")
            n193 = event-data() -> ("CtlRef"=w464:refnum<vi>, "OldVal"=w463:bool)  [unwired: 1 in, 4 out]
            n194 = property class="Bool (严格)"(reference=w464, "Value"=w463) -> ()  [unwired: 1 in, 2 out]
            n195 = call "TMCM351-Step.vi"("错误输入"=w471, "Step"="Step Z", "motor"=w472, "com in"=w473) -> ("错误输出"=w466:errorcluster, "com out"=w467:refnum<visa-resource-name>)  [unwired: 2 in]
          }
          event "X 归0": Value Change {
            w474 = u8 0 items=["x", "y", "z"] ("motor")
            # "判断当前位置，大于0反转，小于0正转"
            n196 = event-data() -> ("CtlRef"=w480:refnum<vi>, "OldVal"=w479:bool)  [unwired: 1 in, 4 out]
            n197 = global write "Verbal.vi" "0位"(u8 1 ("0位")) -> ()
            n198 = disable-structure shown="禁用" {
              disable-tunnel: w478 -> [w489 _]
              disable-tunnel: w475 -> [w488 _]
              disable-tunnel: [w486 _] -> _
              disable-tunnel: [w485 _] -> _
              frame Disabled {
                n199 = local read "当前位置"() -> (w495:string[])
                n200 = Index Array(array=w495, index=0 ("索引")) -> (element=w493:string)
                n201 = Scan From String(format string="X\\t%d" ("格式字符串"), input string=w493) -> (output 1=w491:i32)  [unwired: 3 in, 3 out]
                n202 = global read "Verbal.vi" "speed step"() -> (w487:i32)
                n203 = Greater Than 0?(x=w491) -> (x > 0?=w490:bool)
                n204 = case shown="真" w490 {
                  tunnel: w489 -> [w500 w507]
                  tunnel: w488 -> [w499 w506]
                  tunnel: w487 -> [w498 w505]
                  tunnel: [w497 w504] -> w486
                  tunnel: [w496 w503] -> w485
                  frame False {
                    w502 = u8 0 items=["x", "y", "z"] ("motor")
                    n205 = call "TMCM351-rotate.vi"("motor"=w502, "错误输入"=w499, "正转？"=TRUE, "Speed"=w498, "com in"=w500) -> ("错误输出"=w496:errorcluster, "com out"=w497:refnum<visa-resource-name>)  [unwired: 2 in]
                  }
                  frame True {
                    w509 = u8 0 items=["x", "y", "z"] ("motor")
                    n206 = call "TMCM351-rotate.vi"("motor"=w509, "错误输入"=w506, "正转？"=FALSE, "Speed"=w505, "com in"=w507) -> ("错误输出"=w503:errorcluster, "com out"=w504:refnum<visa-resource-name>)  [unwired: 2 in]
                  }
                }
              }
              frame Enabled {
              }
            }
            n207 = property class="Bool (严格)"(reference=w480, "Value"=w479) -> ()  [unwired: 1 in, 2 out]
            n208 = call "TMCM1021_goRef.vi"("错误输入"=w475, "motor"=w474, "com in"=w478) -> ("错误输出"=w476:errorcluster, "com out"=w477:refnum<visa-resource-name>)
          }
          event "Y 归0": Value Change {
            w512 = u8 1 items=["x", "y", "z"] ("motor")
            n209 = event-data() -> ("CtlRef"=w516:refnum<vi>, "OldVal"=w515:bool)  [unwired: 1 in, 4 out]
            n210 = global write "Verbal.vi" "0位"(u8 2 ("0位")) -> ()
            n211 = property class="Bool (严格)"(reference=w516, "Value"=w515) -> ()  [unwired: 1 in, 2 out]
            n212 = call "TMCM1021_goRef.vi"("错误输入"=w513, "motor"=w512, "com in"=w514) -> ("错误输出"=w510:errorcluster, "com out"=w511:refnum<visa-resource-name>)
            n213 = disable-structure shown="启用" {
              disable-tunnel: w514 -> [w527 _]
              disable-tunnel: w513 -> [w526 _]
              disable-tunnel: [w525 w549] -> w520
              disable-tunnel: [w524 w548] -> w519
              disable-tunnel: w511 -> [_ w549]
              disable-tunnel: w510 -> [_ w548]
              frame Disabled {
                n214 = local read "当前位置"() -> (w523:string[])
                n215 = Index Array(array=w523, index=1 ("索引")) -> (element=w532:string)
                n216 = Scan From String(format string="Y\\t%d" ("格式字符串"), input string=w532) -> (output 1=w530:i32)  [unwired: 3 in, 3 out]
                n217 = global read "Verbal.vi" "speed step"() -> (w528:i32)
                n218 = Greater Than 0?(x=w530) -> (x > 0?=w529:bool)
                n219 = case shown="真" w529 {
                  tunnel: w527 -> [w538 w545]
                  tunnel: w526 -> [w537 w544]
                  tunnel: w528 -> [w536 w543]
                  tunnel: [w535 w542] -> w525
                  tunnel: [w534 w541] -> w524
                  frame False {
                    w540 = u8 1 items=["x", "y", "z"] ("motor")
                    n220 = call "TMCM351-rotate.vi"("motor"=w540, "错误输入"=w537, "正转？"=TRUE, "Speed"=w536, "com in"=w538) -> ("错误输出"=w534:errorcluster, "com out"=w535:refnum<visa-resource-name>)  [unwired: 2 in]
                  }
                  frame True {
                    w547 = u8 1 items=["x", "y", "z"] ("motor")
                    n221 = call "TMCM351-rotate.vi"("motor"=w547, "错误输入"=w544, "正转？"=FALSE, "Speed"=w543, "com in"=w545) -> ("错误输出"=w541:errorcluster, "com out"=w542:refnum<visa-resource-name>)  [unwired: 2 in]
                  }
                }
              }
              frame Enabled {
              }
            }
          }
          event "Z 归0": Value Change {
            w552 = u8 2 items=["x", "y", "z"] ("motor")
            n222 = event-data() -> ("CtlRef"=w556:refnum<vi>, "OldVal"=w555:bool)  [unwired: 1 in, 4 out]
            n223 = global write "Verbal.vi" "0位"(u8 3 ("0位")) -> ()
            n224 = property class="Bool (严格)"(reference=w556, "Value"=w555) -> ()  [unwired: 1 in, 2 out]
            n225 = call "TMCM1021_goRef.vi"("错误输入"=w553, "motor"=w552, "com in"=w554) -> ("错误输出"=w550:errorcluster, "com out"=w551:refnum<visa-resource-name>)
            n226 = disable-structure shown="启用" {
              disable-tunnel: w554 -> [w566 _]
              disable-tunnel: w553 -> [w565 _]
              disable-tunnel: [w564 w587] -> w559
              disable-tunnel: [w563 w588] -> w558
              disable-tunnel: w551 -> [_ w588]
              disable-tunnel: w550 -> [_ w587]
              frame Disabled {
                n227 = local read "当前位置"() -> (w562:string[])
                n228 = Index Array(array=w562, index=2 ("索引")) -> (element=w571:string)
                n229 = Scan From String(format string="Z\\t%d" ("格式字符串"), input string=w571) -> (output 1=w569:i32)  [unwired: 3 in, 3 out]
                n230 = global read "Verbal.vi" "speed step"() -> (w567:i32)
                n231 = Greater Than 0?(x=w569) -> (x > 0?=w568:bool)
                n232 = case shown="真" w568 {
                  tunnel: w566 -> [w577 w584]
                  tunnel: w565 -> [w576 w583]
                  tunnel: w567 -> [w575 w582]
                  tunnel: [w574 w581] -> w563
                  tunnel: [w573 w580] -> w564
                  frame False {
                    w579 = u8 2 items=["x", "y", "z"] ("motor")
                    n233 = call "TMCM351-rotate.vi"("motor"=w579, "错误输入"=w576, "正转？"=TRUE, "Speed"=w575, "com in"=w577) -> ("错误输出"=w573:errorcluster, "com out"=w574:refnum<visa-resource-name>)  [unwired: 2 in]
                  }
                  frame True {
                    w586 = u8 2 items=["x", "y", "z"] ("motor")
                    n234 = call "TMCM351-rotate.vi"("motor"=w586, "错误输入"=w583, "正转？"=FALSE, "Speed"=w582, "com in"=w584) -> ("错误输出"=w580:errorcluster, "com out"=w581:refnum<visa-resource-name>)  [unwired: 2 in]
                  }
                }
              }
              frame Enabled {
              }
            }
          }
          event "X 连续正转": Value Change {
            w595 = u8 0 items=["x", "y", "z"] ("motor")
            n235 = event-data() -> ("CtlRef"=w592:refnum<vi>, "OldVal"=w591:bool)  [unwired: 1 in, 4 out]
            n236 = property class="Bool (严格)"(reference=w592, "Value"=w591) -> ()  [unwired: 1 in, 2 out]
            n237 = global read "Verbal.vi" "speed step"() -> (w597:i32)
            n238 = call "TMCM351-rotate.vi"("motor"=w595, "错误输入"=w598, "正转？"=TRUE, "Speed"=w597, "com in"=w599) -> ("错误输出"=w593:errorcluster, "com out"=w594:refnum<visa-resource-name>)  [unwired: 2 in]
          }
          event "Y 连续正转": Value Change {
            w608 = u8 1 items=["x", "y", "z"] ("motor")
            n239 = event-data() -> ("CtlRef"=w603:refnum<vi>, "OldVal"=w602:bool)  [unwired: 1 in, 4 out]
            n240 = property class="Bool (严格)"(reference=w603, "Value"=w602) -> ()  [unwired: 1 in, 2 out]
            n241 = global read "Verbal.vi" "speed step"() -> (w610:i32)
            n242 = call "TMCM351-rotate.vi"("motor"=w608, "错误输入"=w606, "正转？"=TRUE, "Speed"=w610, "com in"=w607) -> ("错误输出"=w604:errorcluster, "com out"=w605:refnum<visa-resource-name>)  [unwired: 2 in]
          }
          event "Z 连续正转": Value Change {
            w619 = u8 2 items=["x", "y", "z"] ("motor")
            n243 = event-data() -> ("CtlRef"=w614:refnum<vi>, "OldVal"=w613:bool)  [unwired: 1 in, 4 out]
            n244 = property class="Bool (严格)"(reference=w614, "Value"=w613) -> ()  [unwired: 1 in, 2 out]
            n245 = global read "Verbal.vi" "speed step"() -> (w621:i32)
            n246 = call "TMCM351-rotate.vi"("motor"=w619, "错误输入"=w617, "正转？"=TRUE, "Speed"=w621, "com in"=w618) -> ("错误输出"=w615:errorcluster, "com out"=w616:refnum<visa-resource-name>)  [unwired: 2 in]
          }
          event "X连续反转": Value Change {
            w630 = u8 0 items=["x", "y", "z"] ("motor")
            n247 = event-data() -> ("CtlRef"=w625:refnum<vi>, "OldVal"=w624:bool)  [unwired: 1 in, 4 out]
            n248 = property class="Bool (严格)"(reference=w625, "Value"=w624) -> ()  [unwired: 1 in, 2 out]
            n249 = global read "Verbal.vi" "speed step"() -> (w632:i32)
            n250 = call "TMCM351-rotate.vi"("motor"=w630, "错误输入"=w628, "正转？"=FALSE, "Speed"=w632, "com in"=w629) -> ("错误输出"=w626:errorcluster, "com out"=w627:refnum<visa-resource-name>)  [unwired: 2 in]
          }
          event "Y 连续反转": Value Change {
            w642 = u8 1 items=["x", "y", "z"] ("motor")
            n251 = event-data() -> ("CtlRef"=w636:refnum<vi>, "OldVal"=w635:bool)  [unwired: 1 in, 4 out]
            n252 = property class="Bool (严格)"(reference=w636, "Value"=w635) -> ()  [unwired: 1 in, 2 out]
            n253 = global read "Verbal.vi" "speed step"() -> (w643:i32)
            n254 = call "TMCM351-rotate.vi"("motor"=w642, "错误输入"=w639, "正转？"=FALSE, "Speed"=w643, "com in"=w640) -> ("错误输出"=w637:errorcluster, "com out"=w638:refnum<visa-resource-name>)  [unwired: 2 in]
          }
          event "Z 连续反转": Value Change {
            w652 = u8 2 items=["x", "y", "z"] ("motor")
            n255 = event-data() -> ("CtlRef"=w647:refnum<vi>, "OldVal"=w646:bool)  [unwired: 1 in, 4 out]
            n256 = property class="Bool (严格)"(reference=w647, "Value"=w646) -> ()  [unwired: 1 in, 2 out]
            n257 = global read "Verbal.vi" "speed step"() -> (w654:i32)
            n258 = call "TMCM351-rotate.vi"("motor"=w652, "错误输入"=w650, "正转？"=FALSE, "Speed"=w654, "com in"=w651) -> ("错误输出"=w648:errorcluster, "com out"=w649:refnum<visa-resource-name>)  [unwired: 2 in]
          }
          event "X jog": Value Change {
            w658 = u8 0 items=["x", "y", "z"] ("motor")
            n259 = event-data() -> ("CtlRef"=w664:refnum<vi>, "OldVal"=w663:bool)  [unwired: 1 in, 4 out]
            n260 = property class="Bool (严格)"(reference=w664, "Value"=w663) -> ()  [unwired: 1 in, 2 out]
            n261 = local read "X设定位置"() -> (w657:i32)
            n262 = call "TMCM351-goJog.vi"("错误输入"=w661, "step in"=w657, "motor"=w658, "com in"=w662) -> ("错误输出"=w659:errorcluster, "com out"=w660:refnum<visa-resource-name>)  [unwired: 2 in]
          }
          event "Yjog": Value Change {
            w670 = u8 1 items=["x", "y", "z"] ("motor")
            n263 = event-data() -> ("CtlRef"=w674:refnum<vi>, "OldVal"=w673:bool)  [unwired: 1 in, 4 out]
            n264 = property class="Bool (严格)"(reference=w674, "Value"=w673) -> ()  [unwired: 1 in, 2 out]
            n265 = local read "Y设定位置"() -> (w669:i32)
            n266 = call "TMCM351-goJog.vi"("错误输入"=w671, "step in"=w669, "motor"=w670, "com in"=w672) -> ("错误输出"=w667:errorcluster, "com out"=w668:refnum<visa-resource-name>)  [unwired: 2 in]
          }
          event "Zjog": Value Change {
            w680 = u8 2 items=["x", "y", "z"] ("motor")
            n267 = event-data() -> ("CtlRef"=w684:refnum<vi>, "OldVal"=w683:bool)  [unwired: 1 in, 4 out]
            n268 = property class="Bool (严格)"(reference=w684, "Value"=w683) -> ()  [unwired: 1 in, 2 out]
            n269 = local read "Z设定位置"() -> (w679:i32)
            n270 = call "TMCM351-goJog.vi"("错误输入"=w681, "step in"=w679, "motor"=w680, "com in"=w682) -> ("错误输出"=w677:errorcluster, "com out"=w678:refnum<visa-resource-name>)  [unwired: 2 in]
          }
          event "P1jog": Value Change {
            n271 = event-data() -> ("CtlRef"=w696:refnum<vi>, "OldVal"=w695:bool)  [unwired: 1 in, 4 out]
            n272 = property class="Bool (严格)"(reference=w696, "Value"=w695) -> ()  [unwired: 1 in, 2 out]
            n273 = global read "Verbal.vi" "Device Address"() -> (w692:i32)
            n274 = local read "P1设定位置"() -> (w690:i32)
            n275 = global read "Verbal.vi" "DeviceKey"() -> (w693:string)
            n276 = call "AbsoluteMove.vi"("CmdLib In"=w694, "DeviceKey In"=w693, "Device Address In"=w692, "Motor"=1, "Target Pos"=w690, "error in (no error)"=w689) -> ("CmdLib Out"=w688:refnum<k24>, "error out"=w687:errorcluster)  [unwired: 10 in, 2 out]
          }
          event "P2 jog": Value Change {
            n277 = event-data() -> ("CtlRef"=w708:refnum<vi>, "OldVal"=w707:bool)  [unwired: 1 in, 4 out]
            n278 = property class="Bool (严格)"(reference=w708, "Value"=w707) -> ()  [unwired: 1 in, 2 out]
            n279 = global read "Verbal.vi" "Device Address"() -> (w704:i32)
            n280 = global read "Verbal.vi" "DeviceKey"() -> (w705:string)
            n281 = local read "P2设定位置"() -> (w702:i32)
            n282 = call "AbsoluteMove.vi"("CmdLib In"=w706, "DeviceKey In"=w705, "Device Address In"=w704, "Motor"=2, "Target Pos"=w702, "error in (no error)"=w701) -> ("CmdLib Out"=w700:refnum<k24>, "error out"=w699:errorcluster)  [unwired: 10 in, 2 out]
          }
        }
      }
    }
  }
  n283 = call "Shutdown.vi"("error in (no error)"=w3, "CmdLib In"=w4) -> ("error out"=w5:errorcluster, "CmdLib Out"=w6:refnum<k24>)  [unwired: 4 in]
  n284 = call "CloseDevice.vi"("error in"=w5, "CmdLib In"=w6) -> ("error out"=→"error out":errorcluster)  [unwired: 8 in, 1 out]
  n285 = call "TMCM351-STOP.vi"("错误输入"=w13, "motor"=w12, "com in"=w14) -> ("错误输出"=w17:errorcluster, "com out"=w18:refnum<visa-resource-name>)
  n286 = call "TMCM351-STOP.vi"("错误输入"=w17, "motor"=w11, "com in"=w18) -> ("错误输出"=w15:errorcluster, "com out"=w16:refnum<visa-resource-name>)
  n287 = call "TMCM351-STOP.vi"("错误输入"=w15, "motor"=w10, "com in"=w16) -> ("错误输出"=w8:errorcluster, "com out"=w9:refnum<visa-resource-name>)
  n288 = call "TMCM351-STOPexe.vi"("错误输入"=w8, "com in"=w9) -> ("错误输出"=w19:errorcluster, "com out"=w20:refnum<visa-resource-name>)
  n289 = VISA Close(VISA resource name=w20, error in (no error)=w19) -> ()  [unwired: 1 out]
